vi "Input-Y_Graph_RelativeTime.vi"   [LabVIEW 2015, in "GraphPlot.lvlib"]
uses:
  GraphPlot.lvlib
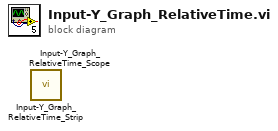
[diagram p0: block diagram]
diagram:
  n1 = call "Input-Y_Graph_RelativeTime_Strip.vi"() -> ()  [unwired: 11 in, 1 out]
  n2 = call "Input-Y_Graph_RelativeTime_Scope.vi"() -> ()  [unwired: 11 in, 1 out]
